vi "Database test.vi"() -> ()   [LabVIEW 2014]
uses:
  <vilib>/drjdpowell/SQLite Library/SQL Statement/SQL Statement.lvclass
  <vilib>/drjdpowell/SQLite Library/SQL Statement/SQL Statement.lvclass/SQL Statement.ctl
  <vilib>/drjdpowell/SQLite Library/SQL Connection/Open (path).vi
  <vilib>/drjdpowell/SQLite Library/SQL Connection/Open (string).vi
  <vilib>/AdvancedString/Path To Command Line String.vi
  <vilib>/drjdpowell/SQLite Library/SQL Statement/Error Message.vi
  <vilib>/drjdpowell/SQLite Library/SQL Statement/Column String.vi
  <vilib>/drjdpowell/SQLite Library/SQL Connection/Connection.lvclass
panel:
  out "error out 3":errorcluster
  out "error out 2":errorcluster
  out "error out":errorcluster
  in  "send query":bool
  out "Get Column:String":string
  out "Valid Statement":bool
  in  "stop":bool
  in  "SQL":string="SELECT test_Name FROM test_table"
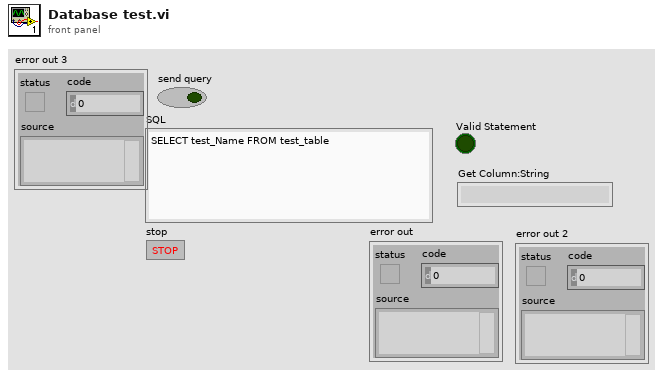
[diagram p1: front panel]
types:
  T1 = enum16{"New or existing", "Existing", "Read only"}
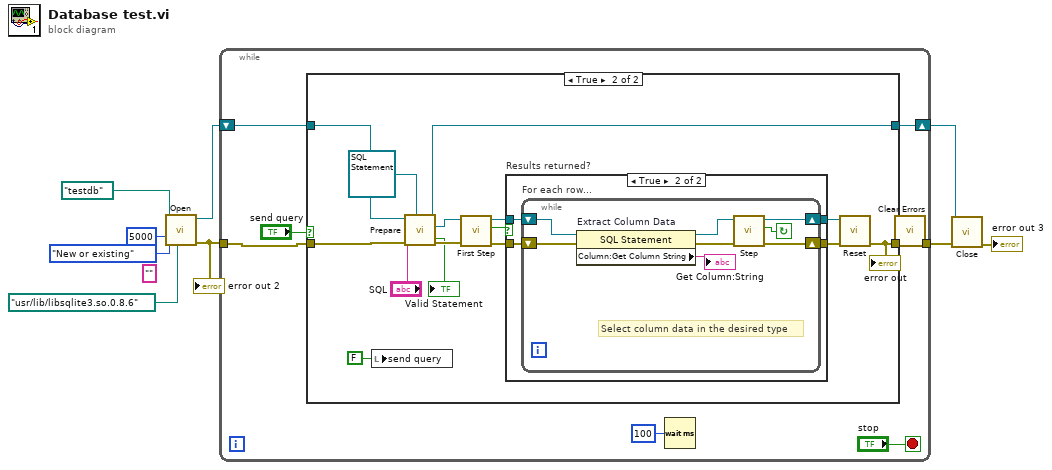
[diagram p0: block diagram]
diagram:
  (unwired) "" ("db file")
  n1 = call-poly <vilib>:"Open.vi"("SQLite Library Path"=path "/usr/lib/libsqlite3.so.0.8.6" ("path"), "File Option"=T1."New or existing", "busy timeout (ms)"=5000, "db file"=path "/testdb") -> ("error out"=w6:errorcluster, "SQLite Connection out"=w7:refnum<class "Connection.lvclass">)  [unwired: 6 in]
  "error out 2" <- w6
  n2 = while {
    shift-right: [w15] -> w5
    shift-left: w7 -> [w17]
    tunnel: w6 -> [w16]
    tunnel: [w10] -> w4
    stop <- "stop" stop-if-true
    n3 = case shown="True" "send query" {
      tunnel: w17 -> [w19 w29]
      tunnel: w16 -> [w18 w28]
      tunnel: [w19 w25] -> w15
      tunnel: [w18 w24] -> w14
      frame False {
      }
      frame True {
        n4 = local write "send query"(FALSE ("send query")) -> ()
        n5 = call <vilib>:"Prepare.vi"("SQL Statement type"=refnum<class "SQL Statement.lvclass"> refnum, "error in (no error)"=w28, "SQL"="SQL", "SQLite Connection in"=w29) -> ("error out"=w26:errorcluster, "SQL Statement out"=w27:refnum<class "SQL Statement.lvclass">, "SQLite Connection out"=w25:refnum<class "Connection.lvclass">, "Valid Statement"=→"Valid Statement":bool)  [unwired: 3 in, 1 out]
        n6 = call <vilib>:"First Step.vi"("error in (no error)"=w26, "SQL Statement in"=w27) -> ("error out"=w31:errorcluster, "Row returned"=w30:bool, "SQL Statement out"=w32:refnum<class "SQL Statement.lvclass">)  [unwired: 7 in]
        n7 = case "Results returned?" shown="True" w30 {
          tunnel: [w36 w40] -> w33
          tunnel: [w35 w39] -> w34
          tunnel: w32 -> [w36 w38]
          tunnel: w31 -> [w35 w37]
          frame False {
          }
          frame True {
            n8 = while "For each row..." {
              shift-right: [w47] -> w40
              shift-left: w38 -> [w44]
              shift-right: [w45] -> w39
              shift-left: w37 -> [w43]
              stop <- w42 continue-if-true
              # "Select column data in the desired type"
              n9 = property on="Extract Column Data" class="SQL Statement"(reference=w44, error in=w43) -> (reference out=w48:refnum<class "SQL Statement.lvclass">, error out=w46:errorcluster, "Column:Get Column String"=→"Get Column:String":string)
              n10 = call <vilib>:"Step.vi"("error in (no error)"=w46, "SQL Statement in"=w48) -> ("error out"=w45:errorcluster, "Row returned"=w42:bool, "SQL Statement out"=w47:refnum<class "SQL Statement.lvclass">)  [unwired: 7 in]
            }
          }
        }
        n11 = call <vilib>:"Reset.vi"("error in (no error)"=w34, "SQL Statement in"=w33) -> ("error out"=w24:errorcluster)  [unwired: 8 in, 1 out]
        "error out" <- w24
      }
    }
    n12 = Wait (ms)(milliseconds to wait=u32 100) -> ()  [unwired: 1 out]
    n13 = call <vilib>:"Clear Errors.vi"("error in (no error)"=w14) -> ("error out"=w10:errorcluster)  [unwired: 5 in, 1 out]
  }
  n14 = call-dynamic "Close.vi"("error in (no error)"=w4, "SQLite Connection in"=w5) -> ("error out"=→"error out 3":errorcluster)  [unwired: 9 in]
